vi "image shift (SubVI).vi"(9 "v shift":i32, 10 "h shift":i32, 11 "Array in":u16[][](array[numeric])) -> (3 "Array out":u16[][](array[numeric]))   [LabVIEW 2024]
uses:
  <vilib>/vision/NI_Vision_Development_Module.lvlib
panel:
  out "x-y":dbl=0.0004460000000108266
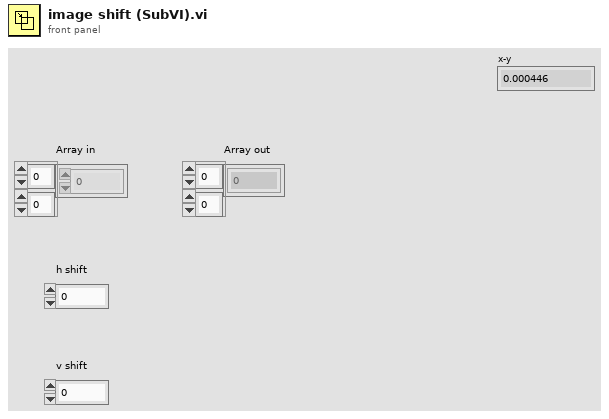
[diagram p1: front panel]
types:
  T1 = typedef "Image Type" = u32
  T2 = typedef "IMAQ Image.ctl" = refnum<image>
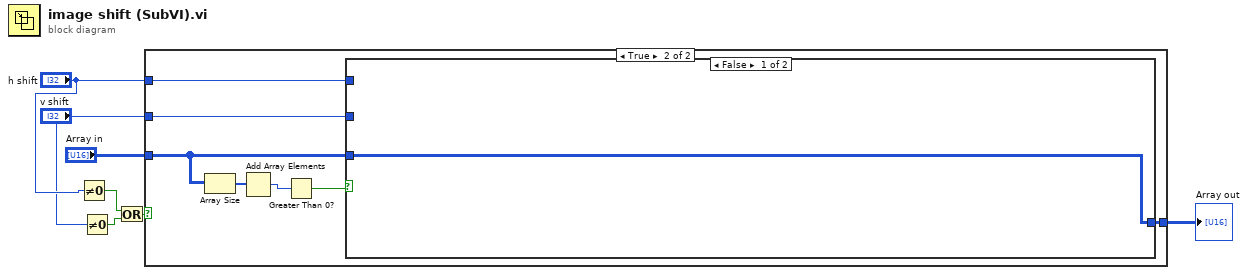
[diagram p0: block diagram]
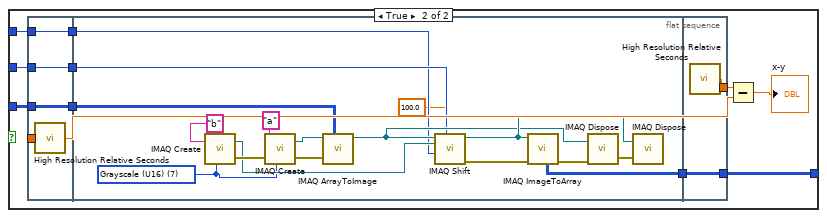
[diagram p3: hidden frame]
diagram:
  n1 = Not Equal To 0?(x="h shift") -> (x != 0?=w2:bool)
  n2 = Not Equal To 0?(x="v shift") -> (x != 0?=w1:bool)
  n3 = Or(x=w2, y=w1) -> (x .or. y?=w5:bool)
  n4 = case shown="True" w5 {
    tunnel: "Array in" -> [w8 w12]
    tunnel: [w8 w15] -> w6
    tunnel: "v shift" -> [_ w14]
    tunnel: "h shift" -> [_ w13]
    frame False {
    }
    frame True {
      n5 = Array Size(array=w12) -> (size(s)=w11:i32[])
      n6 = Add Array Elements(numeric array=w11) -> (sum=w10:i32)
      n7 = Greater Than 0?(x=w10) -> (x > 0?=w9:bool)
      n8 = case shown="False" w9 {
        tunnel: [w16 w23] -> w15
        tunnel: w14 -> [_ w22]
        tunnel: w13 -> [_ w21]
        tunnel: w12 -> [w16 w17]
        frame False {
        }
        frame True {
          n9 = flat-sequence {
            tunnel: w21 -> [w29]
            tunnel: w22 -> [w30]
            tunnel: w17 -> [w31]
            tunnel: [w31] -> w27
            tunnel: [w30] -> w26
            tunnel: [w29] -> w25
            tunnel: [w28] -> w19
            tunnel: w27 -> [w36]
            tunnel: w26 -> [w34]
            tunnel: w25 -> [w33]
            tunnel: [w35] -> w24
            tunnel: [w50] -> w23
            tunnel: w24 -> [w50]
            tunnel: [w49] -> w20
            frame #0 {
              n10 = call <vilib>:"High Resolution Relative Seconds.vi"() -> ("relative seconds"=w28:dbl)
            }
            frame #1 {
              w37 = T1 7 items=["Grayscale (U8)", "Grayscale (I16)", "Grayscale (SGL)", "Complex (CSG)", "RGB (U32)", "HSL (U32)", "RGB (U64)", "Grayscale (U16)"] ("Image Type")
              n11 = call "IMAQ Create"("Image Name"="b", "Image Type"=w37) -> ("New Image"=w42:T2, "error out"=w46:errorcluster)  [unwired: 3 in]
              n12 = call "IMAQ Create"("Image Name"="a", "Image Type"=w37, "error in (no error)"=w46) -> ("New Image"=w47:T2, "error out"=w48:errorcluster)  [unwired: 2 in]
              n13 = call "IMAQ ArrayToImage"("Image Pixels (U16)"=w36, "error in (no error)"=w48, "Image"=w47) -> ("Image Out"=w40:T2)  [unwired: 7 in, 1 out]
              n14 = call "IMAQ Shift"("YOffset"=w34, "Replace Value"=sgl 100.0, "XOffset"=w33, "Image Dst"=w42, "Image Src"=w40) -> ("error out"=w39:errorcluster, "Image Dst Out"=w41:T2)  [unwired: 5 in]
              n15 = call "IMAQ ImageToArray"("error in (no error)"=w39, "Image"=w41) -> ("Image Pixels (U16)"=w35:u16[][], "error out"=w38:errorcluster)  [unwired: 2 in, 3 out]
              n16 = call "IMAQ Dispose"("Image"=w40, "error in (no error)"=w38) -> ("error out"=w45:errorcluster)  [unwired: 4 in]
              n17 = call "IMAQ Dispose"("Image"=w41, "error in (no error)"=w45) -> ()  [unwired: 4 in, 1 out]
            }
            frame #2 {
              n18 = call <vilib>:"High Resolution Relative Seconds.vi"() -> ("relative seconds"=w49:dbl)
            }
          }
          n19 = Subtract(x=w20, y=w19) -> (x-y=→"x-y":dbl)
        }
      }
    }
  }
  "Array out" <- w6
